vi "Rectangle Filter.vi"(0 "Aspect Ratio Upper":dbl, 1 "Index Value":i32, 2 "Lower Limits":dbl[](array[numeric]), 3 "Scored Particle Info":T1(array[cluster]), 4 "Left":bool) -> (5 "Index of Top Rectangle":i32)   [LabVIEW 2013]
panel:
  # "This VI searches through the rectangls found and\nfinds the highest rectange that meets the filtering \nconidtions Left (Right) input required as the cameras \nare rotated 90 degrees in different directions.\n\nPresent Conditions:\nAspect Ratio (Width/Height) (upper and lower limits) \nRectangle Coverage\nX Edge Strength\nY Edge Strength"
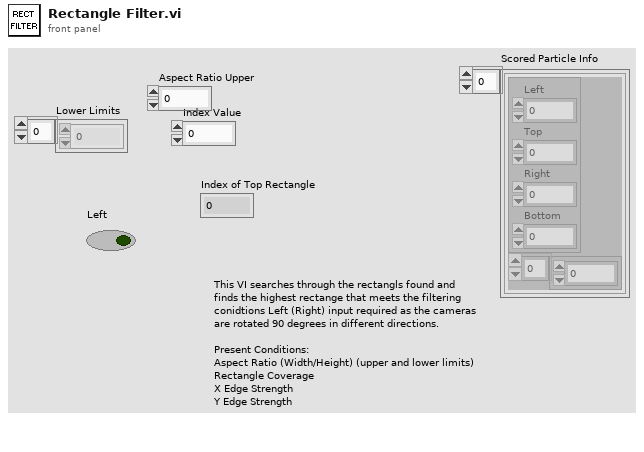
[diagram p1: front panel]
types:
  T1 = cluster{cluster{"Left":dbl, "Top":dbl, "Right":dbl, "Bottom":dbl}, dbl[]}[]
  T2 = cluster{cluster{"Left":dbl, "Top":dbl, "Right":dbl, "Bottom":dbl}, dbl[]}
  T3 = cluster{"Left":dbl, "Top":dbl, "Right":dbl, "Bottom":dbl}
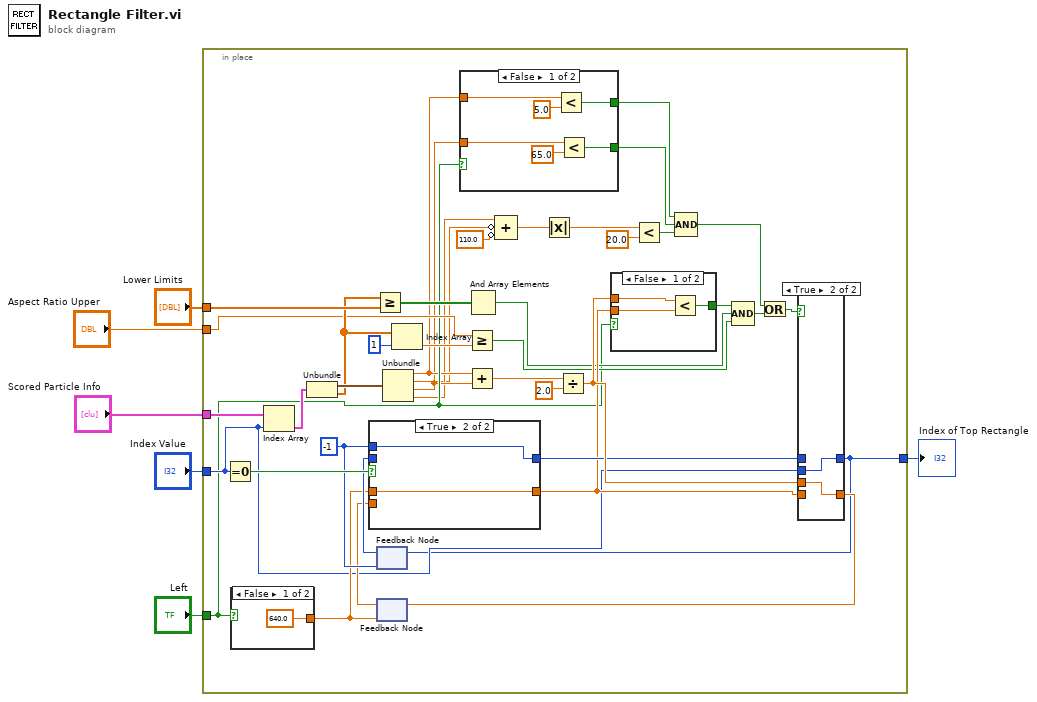
[diagram p0: block diagram]
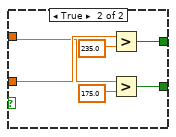
[diagram p2: hidden frame]
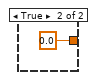
[diagram p3: hidden frame]
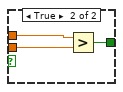
[diagram p4: hidden frame]
diagram:
  n1 = in-place {
    in-place-border: "Scored Particle Info" -> [w33]
    in-place-border: "Index Value" -> [w32]
    in-place-border: [w31] -> w4
    in-place-border: "Lower Limits" -> [w28]
    in-place-border: "Aspect Ratio Upper" -> [w23]
    in-place-border: "Left" -> [w14]
    w40 = -1 ("y")
    n2 = Equal To 0?(x=w32) -> (x = 0?=w41:bool)
    n3 = case shown="False" w14 {
      tunnel: [640.0 ("y") 0.0 ("y")] -> w36
      frame False {
      }
      frame True {
      }
    }
    n4 = Index Array(array=w33, index=w32) -> (element=w46:T2)
    n5 = Unbundle(w46) -> (w34:T3, w26:dbl[])
    n6 = Greater Or Equal?(x=w26, y=w28) -> (x >= y?=w27:bool[])
    n7 = feedback #1(w40) -> (w39:i32)
    n8 = feedback #2(w36) -> (w37:dbl)
    n9 = case shown="True" w41 {
      tunnel: w40 -> [_ w70]
      tunnel: [w68 w70] -> w38
      tunnel: w39 -> [w68 _]
      tunnel: w37 -> [w67 _]
      tunnel: [w67 w69] -> w35
      tunnel: w36 -> [_ w69]
      frame False {
      }
      frame True {
      }
    }
    n10 = Unbundle(w34) -> ("Left"=w13:dbl, "Top"=w10:dbl, "Right"=w12:dbl, "Bottom"=w11:dbl)
    n11 = Index Array(array=w26, index=1) -> (element=w24:dbl)
    n12 = case shown="False" w14 {
      tunnel: w13 -> [w52 w53]
      tunnel: w12 -> [w49 w54]
      tunnel: [w48 w55] -> w16
      tunnel: [w47 w56] -> w15
      frame False {
        n13 = Less?(x=w52, y=5.0) -> (x < y?=w47:bool)
        n14 = Less?(x=w49, y=65.0) -> (x < y?=w48:bool)
      }
      frame True {
        n15 = Greater?(x=w54, y=235.0) -> (0:w56:bool)
        n16 = Greater?(x=w53, y=175.0) -> (0:w55:bool)
      }
    }
    n17 = Greater Or Equal?(x=w23, y=w24) -> (x >= y?=w22:bool)
    n18 = Add(x=w13, y=w12) -> (x+y=w45:dbl)
    n19 = And Array Elements(Boolean array=w27) -> (logical AND=w29:bool)
    n20 = Compound Arithmetic op=ADD(w11, invert w10, invert 110.0 ("value")) -> (w20:dbl)
    n21 = Absolute Value(x=w20) -> (abs(x)=w19:dbl)
    n22 = Divide(x=w45, y=2.0) -> (x/y=w43:dbl)
    n23 = case shown="False" w14 {
      tunnel: w43 -> [w61 w66]
      tunnel: w35 -> [w62 w65]
      tunnel: [w63 w64] -> w30
      frame False {
        n24 = Less?(x=w61, y=w62) -> (x < y?=w63:bool)
      }
      frame True {
        n25 = Greater?(x=w66, y=w65) -> (0:w64:bool)
      }
    }
    n26 = Less?(x=w19, y=20.0) -> (x < y?=w17:bool)
    n27 = Compound Arithmetic op=AND(w15, w16, w17) -> (w9:bool)
    n28 = Compound Arithmetic op=AND(w30, w29, w22) -> (w8:bool)
    n29 = Or(x=w9, y=w8) -> (x .or. y?=w7:bool)
    n30 = case shown="True" w7 {
      tunnel: [w72 w74] -> w42
      tunnel: w43 -> [_ w74]
      tunnel: w35 -> [w72 _]
      tunnel: w38 -> [w71 _]
      tunnel: w32 -> [_ w73]
      tunnel: [w71 w73] -> w31
      frame False {
      }
      frame True {
      }
    }
    n31 = feedback-in #1(w31) -> ()
    n32 = feedback-in #2(w42) -> ()
  }
  "Index of Top Rectangle" <- w4
